vi "早癌诊断结果读取.vi"() -> ()   [LabVIEW 2018]
uses:
  <vilib>/Utility/NIReport.llb/Report Type.ctl
  <vilib>/Utility/NIReport.llb/Append Report Text (str wrap).vi
  <vilib>/Utility/NIReport.llb/NI_report.lvclass
  <vilib>/Utility/NIReport.llb/NI_ReportGenerationCore.lvlib
panel:
  in  "报表模板名称":string caption="报表模板名称（必须在“\\报表模板”目录下）"
  in  "保存报告":bool
  in  "内镜初步诊断报告":string
  out "日期：":string
  in  "报告医师":string
  out "图片文件":string
  in  "水平滑动杆 2":dbl(slide) scale=0.0..1171.0
  out "竖直滑动杆 2":cluster{dbl, dbl}(slide)={0.0, 3.1607515657620047}
  out "C扫图像 2":T1(plugin-control)
  in  "路径":path=path "E:/登陆系统重写/待检测文件路径.txt"
  in  "路径 2":path=path "E:/登陆系统重写/保存文件路径.txt"
  in  "水平滑动杆":dbl(slide) scale=0.0..1171.0
  out "竖直滑动杆":cluster{dbl, dbl}(slide)={0.0, 3.1607515657620047}
  out "C扫图像":T1(plugin-control)
  in  "向前按钮":bool
  in  "确定按钮":bool
  in  "待检测文件":path
  in  "保存文件路径":path
  out "检测图片总数":i32
  out "当前图片名称":string
  in  "下一张":bool
  # "ME-NBI内镜图检测"
  # "图像显示"
  # "早癌分割结果："
  # "的"
  # "低级别瘤变LGIN"
  # "非癌区域"
  # "的"
  # "图像文件夹选取"
  # "图像文件夹选取"
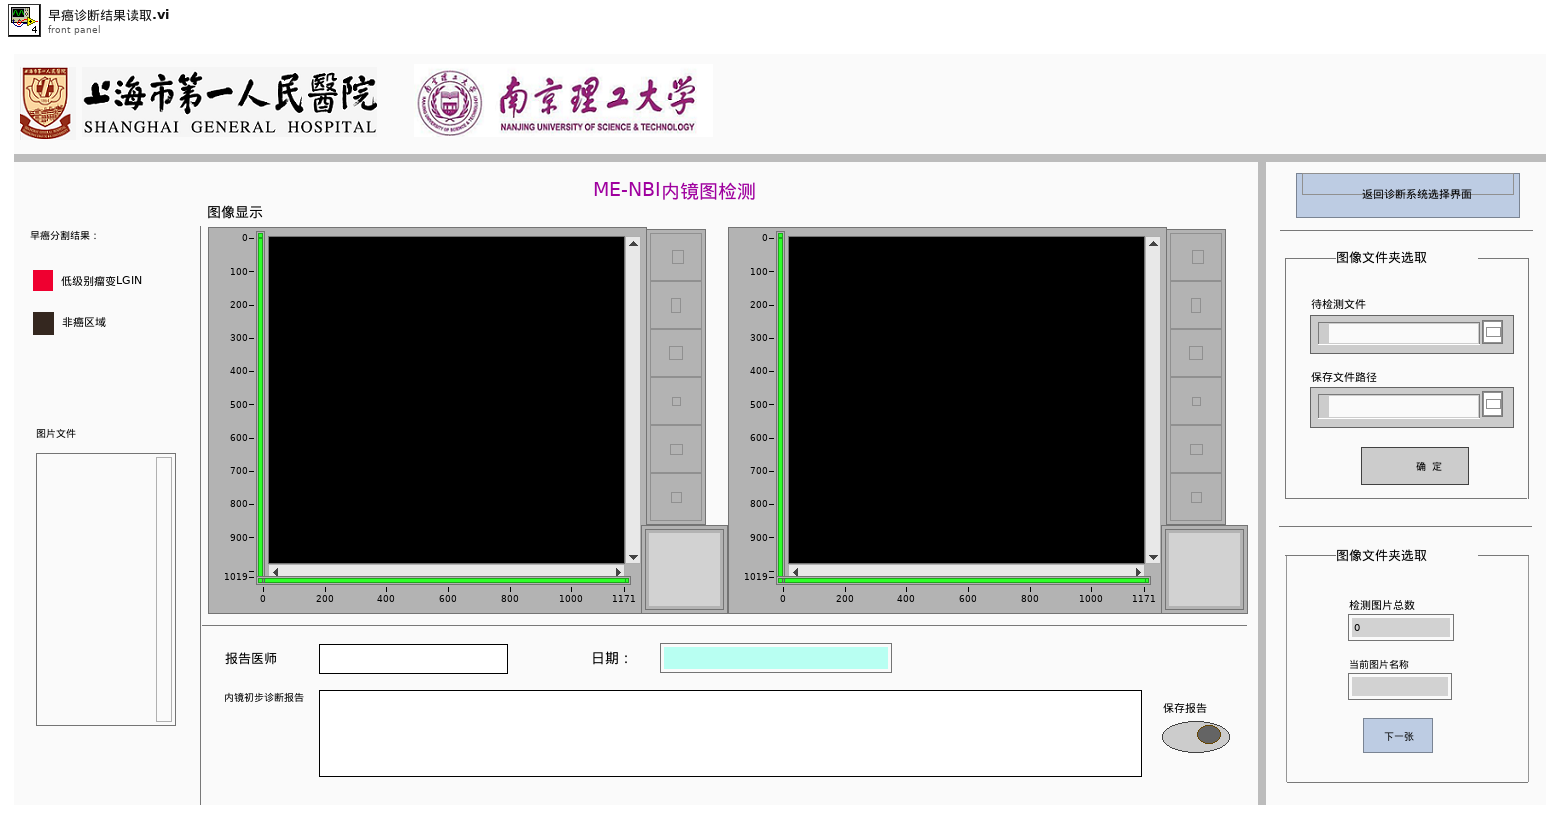
[diagram p1: front panel]
types:
  T1 = typedef "IMAQ Image.ctl" = refnum<image>
  T2 = typedef "Image Type" = u32
  T3 = enum16{"open", "replace", "create", "open or create", "replace or create", "replace or create with confirmation"}
  T4 = enum32{"Invalid", "Standard", "Closed", "Hidden", "Minimized", "Maximized"}
  T5 = enum16{"maximized", "minimized", "normal", "no change"}
  T6 = cluster{"position (Excel)":cluster{"row":i32, "column":i32}, "name (Excel)":string, "bookmark (Word)":string}
  T7 = typedef "NI_ReportGenerationCore.lvlib/Report Type.ctl" = enum16{"HTML", "Word", "Excel"}
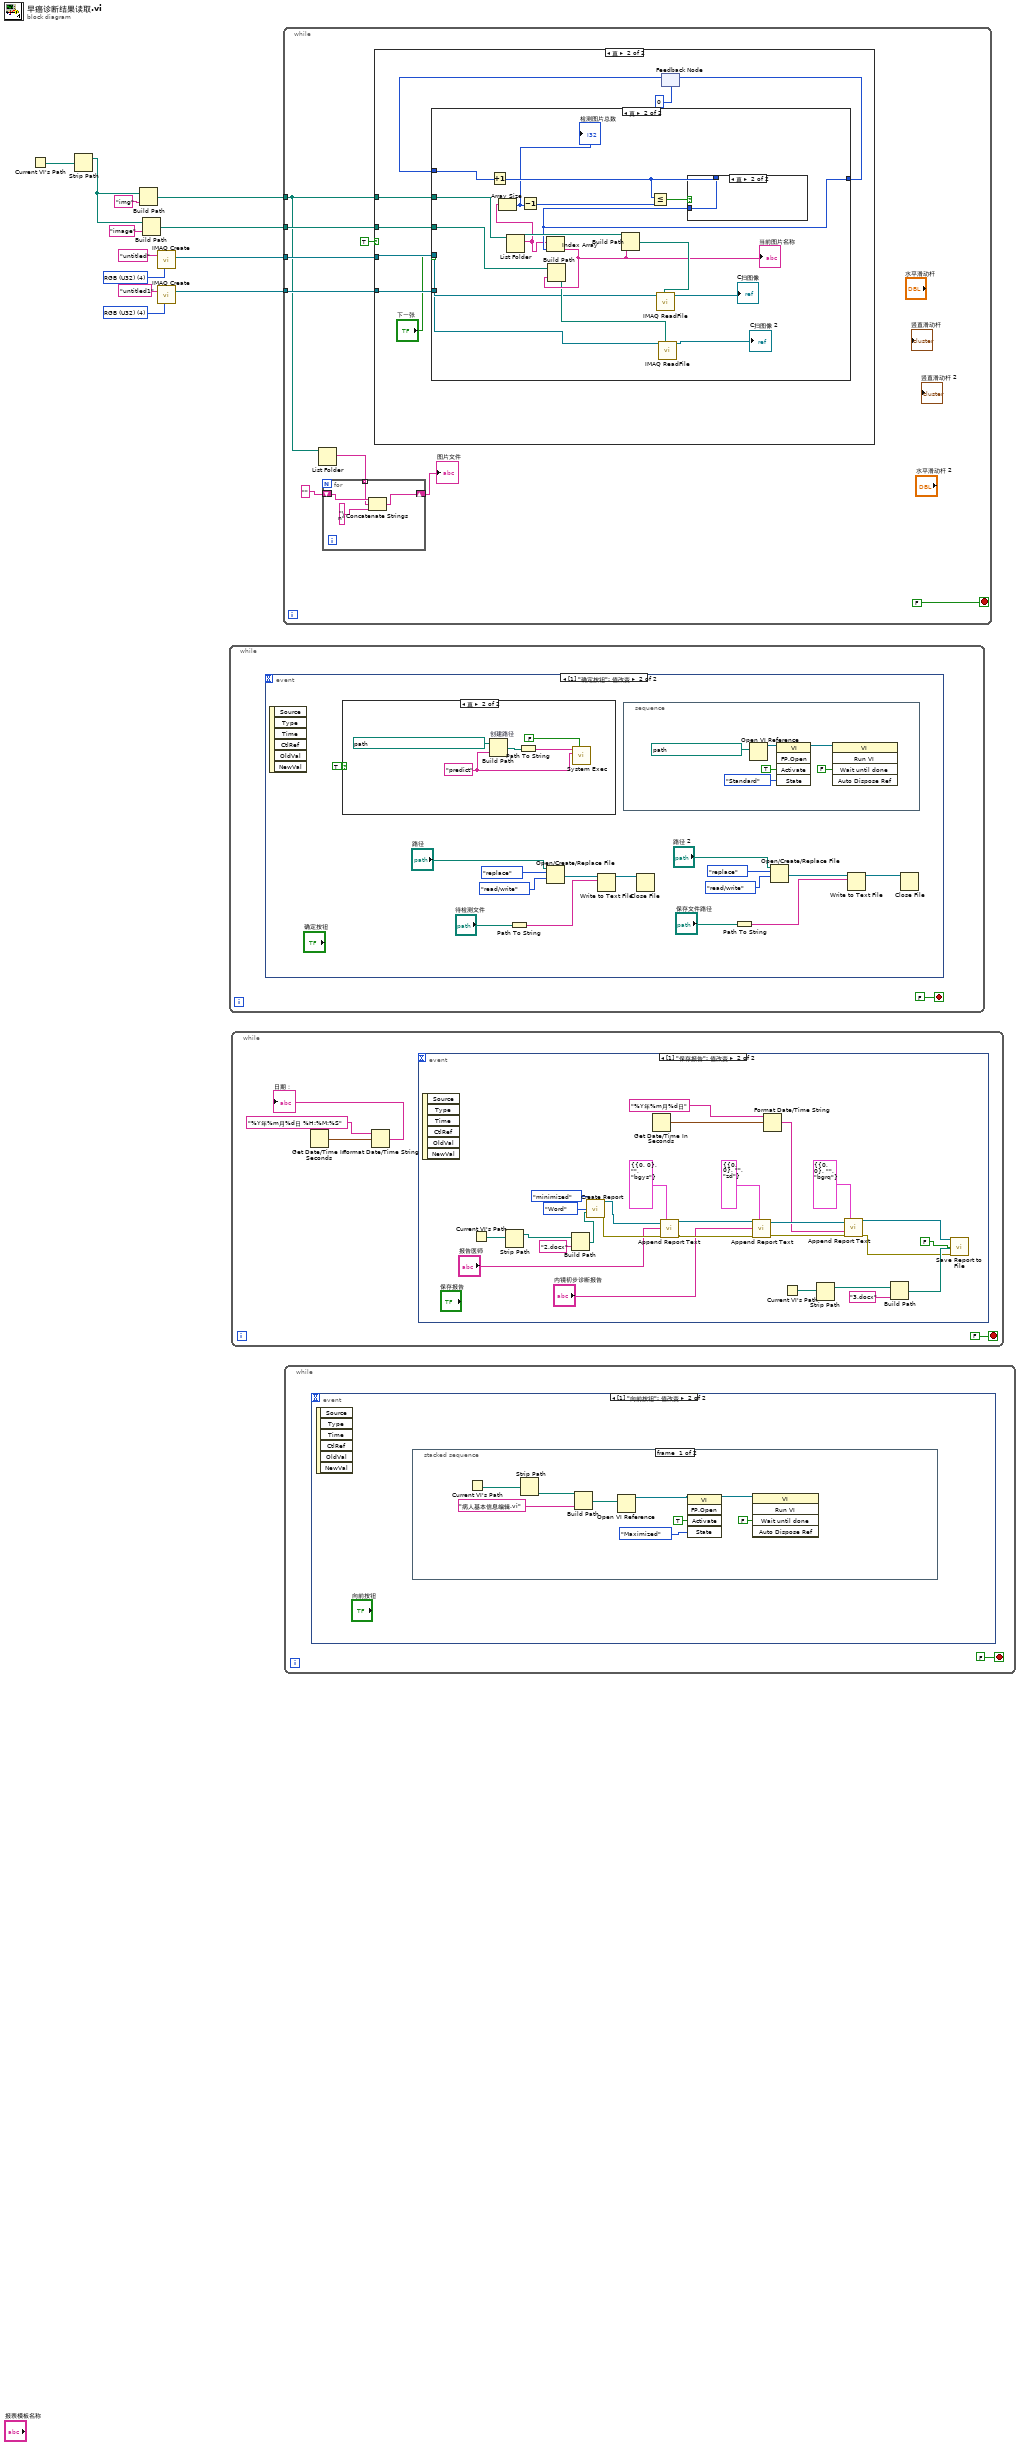
[diagram p0: block diagram]
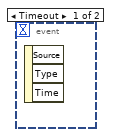
[diagram p2: hidden frame]
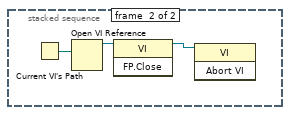
[diagram p3: hidden frame]
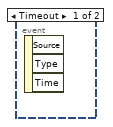
[diagram p4: hidden frame]
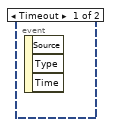
[diagram p5: hidden frame]
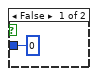
[diagram p9: hidden frame]
diagram:
  w10 = T2 4 items=["Grayscale (U8)", "Grayscale (I16)", "Grayscale (SGL)", "Complex (CSG)", "RGB (U32)", "HSL (U32)", "RGB (U64)", "Grayscale (U16)"] ("Image Type")
  w8 = T2 4 items=["Grayscale (U8)", "Grayscale (I16)", "Grayscale (SGL)", "Complex (CSG)", "RGB (U32)", "HSL (U32)", "RGB (U64)", "Grayscale (U16)"] ("Image Type")
  n1 = Current VI's Path() -> (path=w3:path)
  n2 = Strip Path(path=w3) -> (stripped path=w2:path)  [unwired: 1 out]
  n3 = Build Path(base path=w2, name or relative path="img" ("名称或相对路径")) -> (appended path=w1:path)
  n4 = Build Path(base path=w2, name or relative path="image" ("名称或相对路径")) -> (appended path=w6:path)
  n5 = call "IMAQ Create"("Image Name"="untitled", "Image Type"=w8) -> ("New Image"=w5:T1)  [unwired: 3 in, 1 out]
  n6 = call "IMAQ Create"("Image Name"="untitled1", "Image Type"=w10) -> ("New Image"=w4:T1)  [unwired: 3 in, 1 out]
  n7 = while {
    stop <- FALSE stop-if-true
    n8 = event shown="[1] \"确定按钮\": 值改变" {
      selector: _ -> [_ _]
      dyn-events: _ -> [_ _]
      timeout: _ -> [_ _]
      event Timeout {
        n9 = event-data() -> ()  [unwired: 1 in, 3 out]
      }
      event "确定按钮": Value Change {
        n10 = event-data() -> ()  [unwired: 1 in, 6 out]
        n11 = case shown="真" TRUE {
          frame False {
          }
          frame True {
            w30 = "predict" ("名称或相对路径")
            n12 = Build Path "创建路径"(base path=path "E:/登陆系统重写/早癌诊断/dist/predict" ("基路径"), name or relative path=w30) -> (appended path=w32:path)
            n13 = Path To String(path=w32) -> (string=w33:string)
            n14 = call <vilib>:"System Exec.vi"("wait until completion? (T)"=FALSE, "standard input"=w30, "command line"=w33) -> ()  [unwired: 5 in, 4 out]
          }
        }
        n15 = Path To String(path="待检测文件") -> (string=w23:string)
        n16 = Open/Create/Replace File(file path (use dialog)="路径", operation (0:open)=T3."replace" ("操作(0:open)"), access (0:read/write)=enum16{"read/write", "read-only", "write-only"}."read/write" ("权限(0:read/write)")) -> (refnum out=w25:refnum<file>)  [unwired: 3 in, 2 out]
        n17 = Write to Text File(file (use dialog)=w25, text=w23) -> (refnum out=w24:refnum<file>)  [unwired: 2 in, 2 out]
        n18 = stacked-sequence {
          frame #0 {
            n19 = Open VI Reference(vi path=path "E:/登陆系统重写/进度条.vi" ("VI路径")) -> (vi reference=w39:refnum<vi>)  [unwired: 5 in, 1 out]
            n20 = invoke class="VI" method="FP.Open"(reference=w39, "Activate"=TRUE ("激活？"), "State"=T4."Standard" ("状态")) -> (reference out=w38:refnum<vi>)  [unwired: 2 in, 4 out]
            n21 = invoke class="VI" method="Run VI"(reference=w38, "Wait until done"=FALSE ("结束前等待")) -> ()  [unwired: 3 in, 5 out]
          }
        }
        n22 = Close File(refnum=w24) -> ()  [unwired: 1 in, 2 out]
        n23 = Path To String(path="保存文件路径") -> (string=w19:string)
        n24 = Open/Create/Replace File(file path (use dialog)="路径 2", operation (0:open)=T3."replace" ("操作(0:open)"), access (0:read/write)=enum16{"read/write", "read-only", "write-only"}."read/write" ("权限(0:read/write)")) -> (refnum out=w21:refnum<file>)  [unwired: 3 in, 2 out]
        n25 = Write to Text File(file (use dialog)=w21, text=w19) -> (refnum out=w20:refnum<file>)  [unwired: 2 in, 2 out]
        n26 = Close File(refnum=w20) -> ()  [unwired: 1 in, 2 out]
      }
    }
  }
  n27 = while {
    stop <- FALSE stop-if-true
    n28 = Get Date/Time In Seconds() -> (seconds since 1Jan1904=w41:timestamp)
    n29 = Format Date/Time String(time format string (%c)="%Y年%m月%d日 %H:%M:%S" ("时间格式字符串(%c)"), seconds (now)=w41) -> (date/time string=→"日期：":string)  [unwired: 1 in]
    n30 = event shown="[1] \"保存报告\": 值改变" {
      selector: _ -> [_ _]
      dyn-events: _ -> [_ _]
      timeout: _ -> [_ _]
      event Timeout {
        n31 = event-data() -> ()  [unwired: 1 in, 3 out]
      }
      event "保存报告": Value Change {
        n32 = event-data() -> ()  [unwired: 1 in, 6 out]
        n33 = Current VI's Path() -> (path=w69:path)
        n34 = Strip Path(path=w69) -> (stripped path=w68:path)  [unwired: 1 out]
        n35 = Build Path(base path=w68, name or relative path="2.docx" ("名称或相对路径")) -> (appended path=w70:path)
        n36 = call <vilib>:"Create Report.vi"("window state (normal)"=T5."minimized", "report type"=Report_Type."Word" ("Report Type"), "template (empty)"=w70) -> ("report out"=w67:refnum<class "NI_report.lvclass">, "error out"=w66:errorcluster)  [unwired: 11 in]
        n37 = Get Date/Time In Seconds() -> (seconds since 1Jan1904=w46:timestamp)
        n38 = call-poly <vilib>:"Append Report Text.vi"("report in"=w67, "MS Office parameters"=T6 {"position (Excel)"={"row"=0, "column"=0}, "name (Excel)"="", "bookmark (Word)"="bgys"}, "text"="报告医师", "error in (no error)"=w66) -> ("report out"=w62:refnum<class "NI_report.lvclass">, "error out"=w61:errorcluster)  [unwired: 8 in, 2 out]
        n39 = call-poly <vilib>:"Append Report Text.vi"("report in"=w62, "MS Office parameters"=T6 {"position (Excel)"={"row"=0, "column"=0}, "name (Excel)"="", "bookmark (Word)"="zd"}, "text"="内镜初步诊断报告", "error in (no error)"=w61) -> ("report out"=w58:refnum<class "NI_report.lvclass">, "error out"=w57:errorcluster)  [unwired: 8 in, 2 out]
        n40 = Format Date/Time String(time format string (%c)="%Y年%m月%d日" ("时间格式字符串(%c)"), seconds (now)=w46) -> (date/time string=w44:string)  [unwired: 1 in]
        n41 = Current VI's Path() -> (path=w65:path)
        n42 = Strip Path(path=w65) -> (stripped path=w64:path)  [unwired: 1 out]
        n43 = call-poly <vilib>:"Append Report Text.vi"("report in"=w58, "MS Office parameters"=T6 {"position (Excel)"={"row"=0, "column"=0}, "name (Excel)"="", "bookmark (Word)"="bgrq"}, "text"=w44, "error in (no error)"=w57) -> ("report out"=w56:refnum<class "NI_report.lvclass">, "error out"=w55:errorcluster)  [unwired: 8 in, 2 out]
        n44 = Build Path(base path=w64, name or relative path="3.docx" ("名称或相对路径")) -> (appended path=w63:path)
        n45 = call-dynamic "Save Report to File.vi"("report in"=w56, "report file path"=w63, "prompt to replace? (F)"=FALSE, "error in (no error)"=w55) -> ()  [unwired: 10 in, 2 out]
      }
    }
  }
  n46 = while {
    tunnel: w1 -> [w74]
    tunnel: w6 -> [w78]
    tunnel: w5 -> [w77]
    tunnel: w4 -> [w76]
    stop <- FALSE stop-if-true
    n47 = List Folder(path=w74) -> (filenames=w72:string[])  [unwired: 3 in, 3 out]
    n48 = for {
      shift-right: [w83] -> w71
      shift-left: "" -> [w82]
      tunnel: w72 -> [w80] mode=indexing
      n49 = Concatenate Strings(w82, w80, "\n" ("字符串")) -> (w83:string)
    }
    "图片文件" <- w71
    n50 = case shown="真" TRUE {
      tunnel: w74 -> [_ w90]
      tunnel: w78 -> [_ w89]
      tunnel: w77 -> [_ w88]
      tunnel: w76 -> [_ w87]
      frame False {
      }
      frame True {
        n51 = feedback #1(0) -> (w85:i32)
        n52 = case shown="真" "下一张" {
          tunnel: w90 -> [_ w105]
          tunnel: w89 -> [_ w104]
          tunnel: w88 -> [_ w103]
          tunnel: w87 -> [_ w102]
          tunnel: w85 -> [w92 w101]
          tunnel: [w92 w98] -> w84
          frame False {
          }
          frame True {
            n53 = Increment(x=w101) -> (x+1=w99:i32)
            n54 = List Folder ("罗列文件夹")(path=w105) -> (path out=w109:path, filenames=w93:string[])  [unwired: 3 in, 2 out]
            n55 = Array Size(array=w93) -> (size(s)=w96:i32)
            "检测图片总数" <- w96
            n56 = Decrement(x=w96) -> (x-1=w97:i32)
            n57 = Less Or Equal?(x=w99, y=w97) -> (x <= y?=w100:bool)
            n58 = case shown="真" w100 {
              tunnel: [0 w111] -> w98
              tunnel: w99 -> [_ w111]
              frame False {
              }
              frame True {
              }
            }
            n59 = Index Array(array=w93, index=w98) -> (element=w107:string)
            "当前图片名称" <- w107
            n60 = Build Path(base path=w104, name or relative path=w107) -> (appended path=w106:path)
            n61 = Build Path(base path=w109, name or relative path=w107) -> (appended path=w108:path)
            n62 = call "IMAQ ReadFile"("File Path"=w108, "Image"=w103) -> ("Image Out"=→"C扫图像":T1)  [unwired: 5 in, 4 out]
            n63 = call "IMAQ ReadFile"("File Path"=w106, "Image"=w102) -> ("Image Out"=→"C扫图像 2":T1)  [unwired: 5 in, 4 out]
          }
        }
        n64 = feedback-in #1(w84) -> ()
      }
    }
  }
  n65 = while {
    stop <- FALSE stop-if-true
    n66 = event shown="[1] \"向前按钮\": 值改变" {
      selector: _ -> [_ _]
      dyn-events: _ -> [_ _]
      timeout: _ -> [_ _]
      event Timeout {
        n67 = event-data() -> ()  [unwired: 1 in, 3 out]
      }
      event "向前按钮": Value Change {
        n68 = event-data() -> ()  [unwired: 1 in, 6 out]
        n69 = stacked-sequence {
          frame #0 {
            n70 = Current VI's Path() -> (path=w119:path)
            n71 = Strip Path(path=w119) -> (stripped path=w120:path)  [unwired: 1 out]
            n72 = Build Path(base path=w120, name or relative path="病人基本信息编辑.vi" ("名称或相对路径")) -> (appended path=w121:path)
            n73 = Open VI Reference(vi path=w121) -> (vi reference=w117:refnum<vi>)  [unwired: 5 in, 1 out]
            n74 = invoke class="VI" method="FP.Open"(reference=w117, "Activate"=TRUE ("激活？"), "State"=T4."Maximized" ("状态")) -> (reference out=w118:refnum<vi>)  [unwired: 2 in, 4 out]
            n75 = invoke class="VI" method="Run VI"(reference=w118, "Wait until done"=FALSE ("结束前等待")) -> ()  [unwired: 3 in, 5 out]
          }
          frame #1 {
            n76 = Current VI's Path() -> (path=w124:path)
            n77 = Open VI Reference(vi path=w124) -> (vi reference=w123:refnum<vi>)  [unwired: 5 in, 1 out]
            n78 = invoke class="VI" method="FP.Close"(reference=w123) -> (reference out=w122:refnum<vi>)  [unwired: 2 in, 2 out]
            n79 = invoke class="VI" method="Abort VI"(reference=w122) -> ()  [unwired: 2 in, 3 out]
          }
        }
      }
    }
  }
